vi "MultiListBox.vi"() -> ()   [LabVIEW 2015]
panel:
  in  "Col":i32
  in  "Row":i32
  in  "Multicolumn Listbox":i32(listbox)
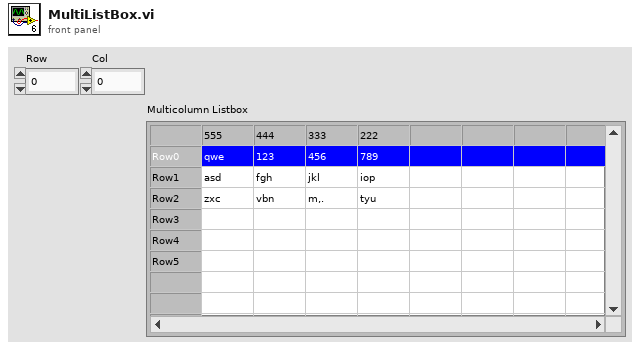
[diagram p1: front panel]
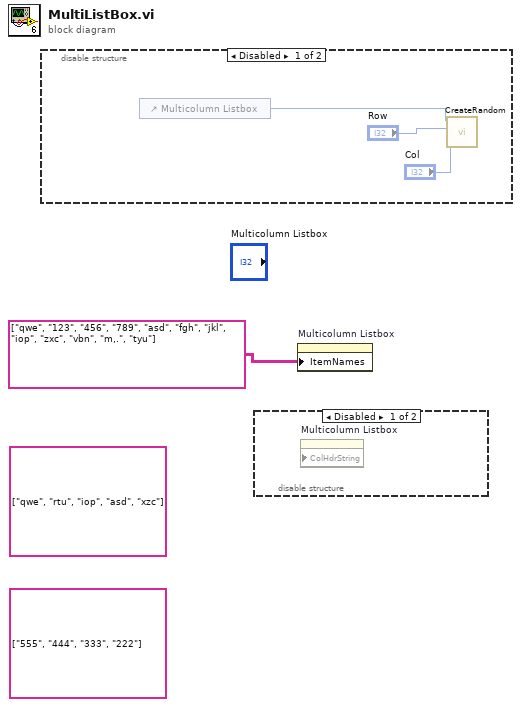
[diagram p0: block diagram]
diagram:
  (unwired) string[] ["555", "444", "333", "222"] ("Column Header Strings[]")
  (unwired) string[] ["qwe", "rtu", "iop", "asd", "xzc"] ("Column Header Strings[]")
  n1 = disable-structure shown="Disabled" {
    frame Disabled {
      n2 = control-ref of="Multicolumn Listbox"() -> (w2:refnum<vi>)
      n3 = call "CreateRandom.vi"("Col"="Col", "Row"="Row", "MCListbox Refnum"=w2) -> ()  [unwired: 8 in, 1 out]
    }
    frame Enabled {
    }
  }
  n4 = disable-structure shown="Disabled" {
    frame Disabled {
      n5 = property on="Multicolumn Listbox" class="MCListbox (strict)" props=["ColHdrString"]() -> ()  [unwired: 3 in, 2 out]
    }
    frame Enabled {
    }
  }
  n6 = property on="Multicolumn Listbox" class="MCListbox (strict)"("ItemNames"=string[][] [["qwe", "123", "456", "789"], ["asd", "fgh", "jkl", "iop"], ["zxc", "vbn", "m,.", "tyu"]]) -> ()  [unwired: 2 in, 2 out]
